vi "ToErrorCluster.vi"(1 "error code":i32 format="%x") -> (0 "error out":errorcluster)   [LabVIEW 2015]
doc: "Translate DAQNavi's error code to labview's error cluster"
uses:
  Windows/System32/AdvLvDaq.dll
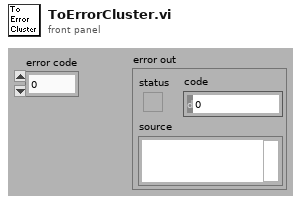
[diagram p1: front panel]
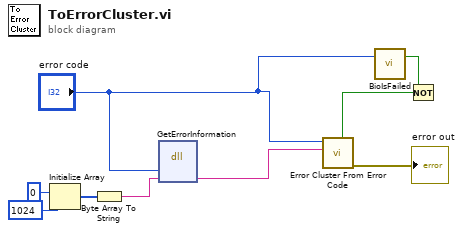
[diagram p0: block diagram]
diagram:
  n1 = Initialize Array(u8 0 ("element"), 1024 ("dimension size")) -> (w2:u8[])
  n2 = Byte Array To String(unsigned byte array=w2) -> (string=w1:string)
  n3 = dll-call lib="C:/Windows/System32/AdvLvDaq.dll" fn="GetErrorInformation"("err"="error code", "info"=w1) -> ("info"=w5:string)  [unwired: 4 in, 3 out]
  n4 = call "BioIsFailed.vi"("ErrorCode"="error code") -> ("IsFailed?"=w8:bool)  [unwired: 2 out]
  n5 = Not(x=w8) -> (.not. x?=w9:bool)
  n6 = call <vilib>:"Error Cluster From Error Code.vi"("is warning? (False)"=w9, "error message (\"\")"=w5, "error code (0)"="error code") -> ("error out"=→"error out":errorcluster)  [unwired: 2 in, 4 out]
